vi "Set Origin To Zero.vi"(8 "error in (no error)":errorcluster, 11 "Pane in":refnum<class "Pane.lvclass">) -> (0 "error out":errorcluster, 3 "Pane out":refnum<class "Pane.lvclass">)   [LabVIEW 2017, in "Pane.lvclass"]
uses:
  Pane.lvclass
  Typedefs/Point--Cluster.ctl
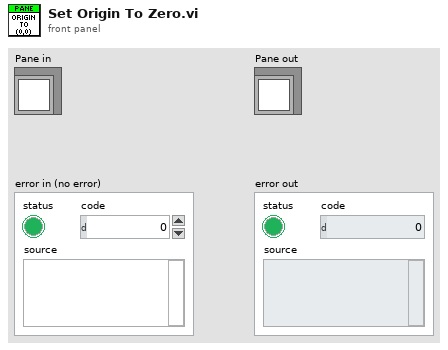
[diagram p1: front panel]
types:
  T1 = typedef "Point--Cluster.ctl" = cluster{"Horizontal":i32, "Vertical":i32}
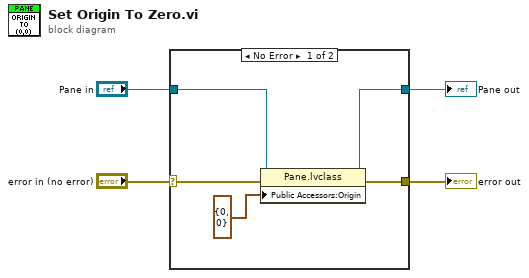
[diagram p0: block diagram]
diagram:
  n1 = case shown="No Error" "error in (no error)" {
    selector: "error in (no error)" -> [w9 w10]
    tunnel: [w8 w10] -> w3
    tunnel: "Pane in" -> [w7 w11]
    tunnel: [w6 w11] -> w1
    frame No Error {
      n2 = property class="Pane.lvclass"(reference=w7, error in=w9, "Public Accessors:Origin"=T1 {"Horizontal"=0, "Vertical"=0} ("Origin")) -> (reference out=w6:refnum<class "Pane.lvclass">, error out=w8:errorcluster)
    }
    frame Error {
    }
  }
  "Pane out" <- w1
  "error out" <- w3
